vi "PWM Config Pane.vi"(6 "_SubPanelMessages":refnum<notifier>, 9 "_myEmbeddedToFrameEvent":T7, 10 "_myEmbedded.Exit":refnum<user-event>, 11 "-Property Bundle":cluster{"Name":string, "Value":variant}[](array[cluster])) -> (1 "_Connection Informations":T1, 2 "_Scripter Input":T9)   [LabVIEW 2021]
doc: "Generates a pulse width modulation (PWM) signal."
uses:
  <vilib>/myRIO/Common/Express VI Framework/xctls/myRIO Channel Name/myRIO Channel Name.xctl
  <vilib>/myRIO/Common/Express VI Framework/typedefs/Config Pane to Framework Ref.ctl
  <vilib>/myRIO/Common/Express VI Framework/typedefs/Data Validate Ref.ctl
  <vilib>/myRIO/Common/Express VI Framework/typedefs/Scripter Input.ctl
  <vilib>/myRIO/Common/Express VI Framework/typedefs/WireThrough Terminal Names.ctl
  <vilib>/myRIO/Common/Express VI Framework/typedefs/Instrument Driver Method Descriptor Array.ctl
  <vilib>/myRIO/Common/Express VI Framework/typedefs/Instrument Driver Method Descriptor.ctl
  <vilib>/myRIO/Common/Express VI Framework/typedefs/Sub Panel Messages.ctl
  <vilib>/myRIO/Common/Express VI Framework/typedefs/Connection Informations.ctl
  <vilib>/myRIO/Common/Instrument Driver Framework/Utilities/typedefs/Channel Types.ctl
  <vilib>/myRIO/Common/Express VI Framework/vis/Express VI Framework Strings Global.vi
panel:
  out "-Channel Details:":string caption="Connection:"
  in  "Duty Cycle:":dbl(slide)=0.5 min=0.0 max=1.0 step=0.01 scale=0.0..1.0
  out "_learnMoreFrequency":string="Detailed information about valid frequencies for this Express VI.\nLearn more"
  in  "_Validate":bool
  in  "Frequency:":dbl=1000.0 min=0.0 max=400000.0
  in  "Frequency Unit":enum16{"Hz", "kHz"}(ring)
  in  "Duty cycle mode":T2(radio) caption="Duty cycle:"
  in  "Frequency mode":T3(radio) caption="Frequency:"
  out "_Output Preview:":dbl[](graph) caption="Output preview:"
  in  "Channel:":u16(xcontrol)
  in  "_Default Alias String":string
  in  "_VI Default Name (Edit and make value default)":string="PWM"
  in  "Name:":string caption="Node name:"
  in  "_WireThrough Info (Edit and make value default)":T4={"WireThrough Top In"="PWM Ref In", "WireThrough Bottom In"="error in (no error)", "WireThrough Top Out"="PWM Ref Out", "WireThrough Bottom Out"="error out"}
  in  "_Template Array (Edit and make value default)":T5=[{"Function Name"="Smart Open", "VI Path"=path "<vilib>/myRIO/Instrument Drivers/Onboard IO/PWM/vis", "Script"=TRUE, "Inputs"=[{"name"="Channel Name", "value"=variant, "Config Pane Only"=TRUE, "Build Array"=FALSE, "Bundle Cluster"=FALSE, "Show Term"=FALSE, "alias"=[], "Required Input"=FALSE}], "Outputs"=[], "VI Class"=enum."Open", "Controls Refs[]"=[], "Inline"=FALSE}, {"Function Name"="Open", "VI Path"=path "<vilib>/myRIO/Instrument Drivers/Onboard IO/PWM/vis", "Script"=FALSE, "Inputs"=[{"name"="Channel Name", "value"=variant, "Config Pane Only"=TRUE, "Build Array"=FALSE, "Bundle Cluster"=FALSE, "Show Term"=FALSE, "alias"=[], "Required Input"=FALSE}], "Outputs"=[], "VI Class"=enum."Open", "Controls Refs[]"=[], "Inline"=FALSE}, {"Function Name"="Set Duty Cycle and Frequency", "VI Path"=path "<vilib>/myRIO/Instrument Drivers/Onboard IO/PWM/vis", "Script"=TRUE, "Inputs"=[{"name"="Duty Cycle", "value"=variant, "Config Pane Only"=FALSE, "Build Array"=FALSE, "Bundle Cluster"=FALSE, "Show Term"=TRUE, "alias"=[], "Required Input"=TRUE}, {"name"="Frequency [Hz]", "value"=variant, "Config Pane Only"=FALSE, "Build Array"=FALSE, "Bundle Cluster"=FALSE, "Show Term"=TRUE, "alias"=[], "Required Input"=TRUE}], "Outputs"=[], "VI Class"=enum."Data", "Controls Refs[]"=[], "Inline"=FALSE}, {"Function Name"="Close", "VI Path"=path "<vilib>/myRIO/Instrument Drivers/Onboard IO/PWM/vis", "Script"=FALSE, "Inputs"=[], "Outputs"=[], "VI Class"=enum."Close", "Controls Refs[]"=[], "Inline"=FALSE}]
  in  "_Test Close":bool
  # "User Visible Area"
  # "NOTE: Tab Order has been set\nfor this Front Panel.\n\nSee Edit>>Set Tabbing Order...\n\nAll controls that are not visible at \nruntime are excluded from Tabbing order\n\nTo exlude a control from context\nhelp prefix its label text with a '-'"
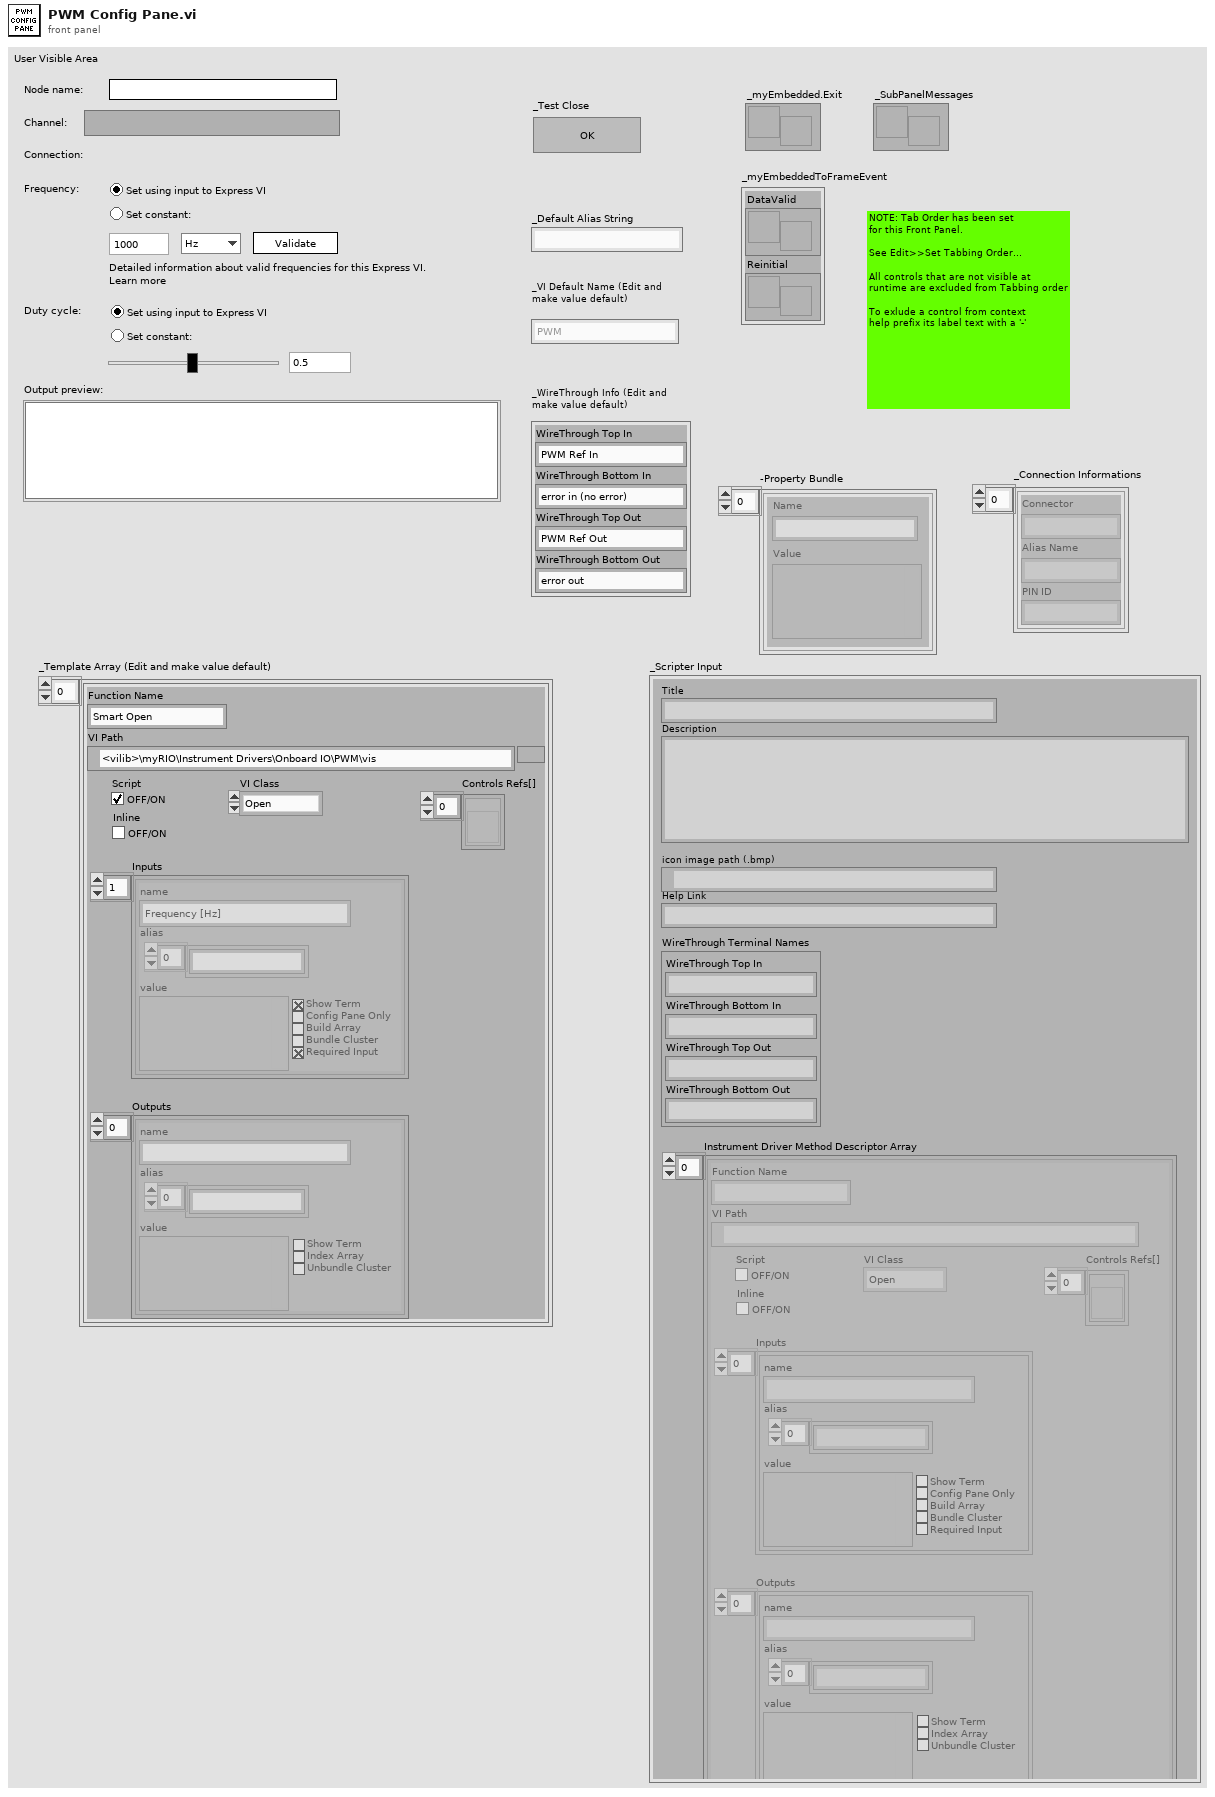
[diagram p1: front panel]
types:
  T1 = typedef "Connection Informations.ctl" = cluster{"Connector":string, "Alias Name":string, "PIN ID":string}[]
  T2 = enum32{"Run-time duty cycle", "Constant duty cycle"}
  T3 = enum32{"Run-time frequency", "Constant frequency"}
  T4 = typedef "WireThrough Terminal Names.ctl" = cluster{"WireThrough Top In":string, "WireThrough Bottom In":string, "WireThrough Top Out":string, "WireThrough Bottom Out":string}
  T5 = typedef "Instrument Driver Method Descriptor Array.ctl" = T6[]
  T6 = typedef "Instrument Driver Method Descriptor.ctl" = cluster{"Function Name":string, "VI Path":path, "Script":bool, "Inputs":cluster{"name":string, "value":variant, "Config Pane Only":bool, "Build Array":bool, "Bundle Cluster":bool, "Show Term":bool, "alias":string[], "Required Input":bool}[], "Outputs":cluster{"name":string, "value":variant, "Show Term":bool, "Index Array":bool, "Unbundle Cluster":bool, "alias":string[]}[], "VI Class":enum16{"Open", "Configure", "Data", "Manage", "Close"}, "Controls Refs[]":refnum<vi>[], "Inline":bool}
  T7 = typedef "Config Pane to Framework Ref.ctl" = cluster{"DataValid":T8, "Reinitial":refnum<user-event>}
  T8 = typedef "Data Validate Ref.ctl" = refnum<user-event>
  T9 = typedef "Scripter Input.ctl" = cluster{"Title":string, "Description":string, "icon image path (.bmp)":path, "Help Link":string, "WireThrough Terminal Names":T4, "Instrument Driver Method Descriptor Array":T5}
  T10 = enum8{"Enabled", "Disabled", "Disabled and Grayed Out"}
  T11 = typedef "Channel Types.ctl" = enum32{"Unknown", "AI", "AO", "DIO - DI", "DIO", "DIO - DO", "I2C", "PWM", "Encoder", "SPI", "UART", "Accelerometer", "DIO - LED", "DIO - Button", "AI (N Samples)", "AudioIn (N Samples)", "AO (N Samples)", "AudioOut (N Samples)", "DI (N Samples)", "DO (N Samples)", "AI IRQ", "DI IRQ", "Timer IRQ", "RSL", "Relay", "CAN", "AI (Continuous)", "AO (Continuous)"}
  T12 = typedef "Channel Info.ctl" = cluster{"Channel Name":string, "Alias":string, "Used?":bool, "Not Support?":bool, "Property Bundle":cluster{"Name":string, "Value":variant}[]}
  T13 = typedef "Sub Panel Messages.ctl" = enum16{"Initialized"}
  T14 = cluster{"Connector":string, "Alias Name":string, "PIN ID":string}
  T15 = cluster{"name":string, "value":variant, "Config Pane Only":bool, "Build Array":bool, "Bundle Cluster":bool, "Show Term":bool, "alias":string[], "Required Input":bool}[]
  T16 = cluster{"name":string, "value":variant, "Config Pane Only":bool, "Build Array":bool, "Bundle Cluster":bool, "Show Term":bool, "alias":string[], "Required Input":bool}
  T17 = cluster{"Connector":string, "Alias Name":string, "PIN ID":string}[]
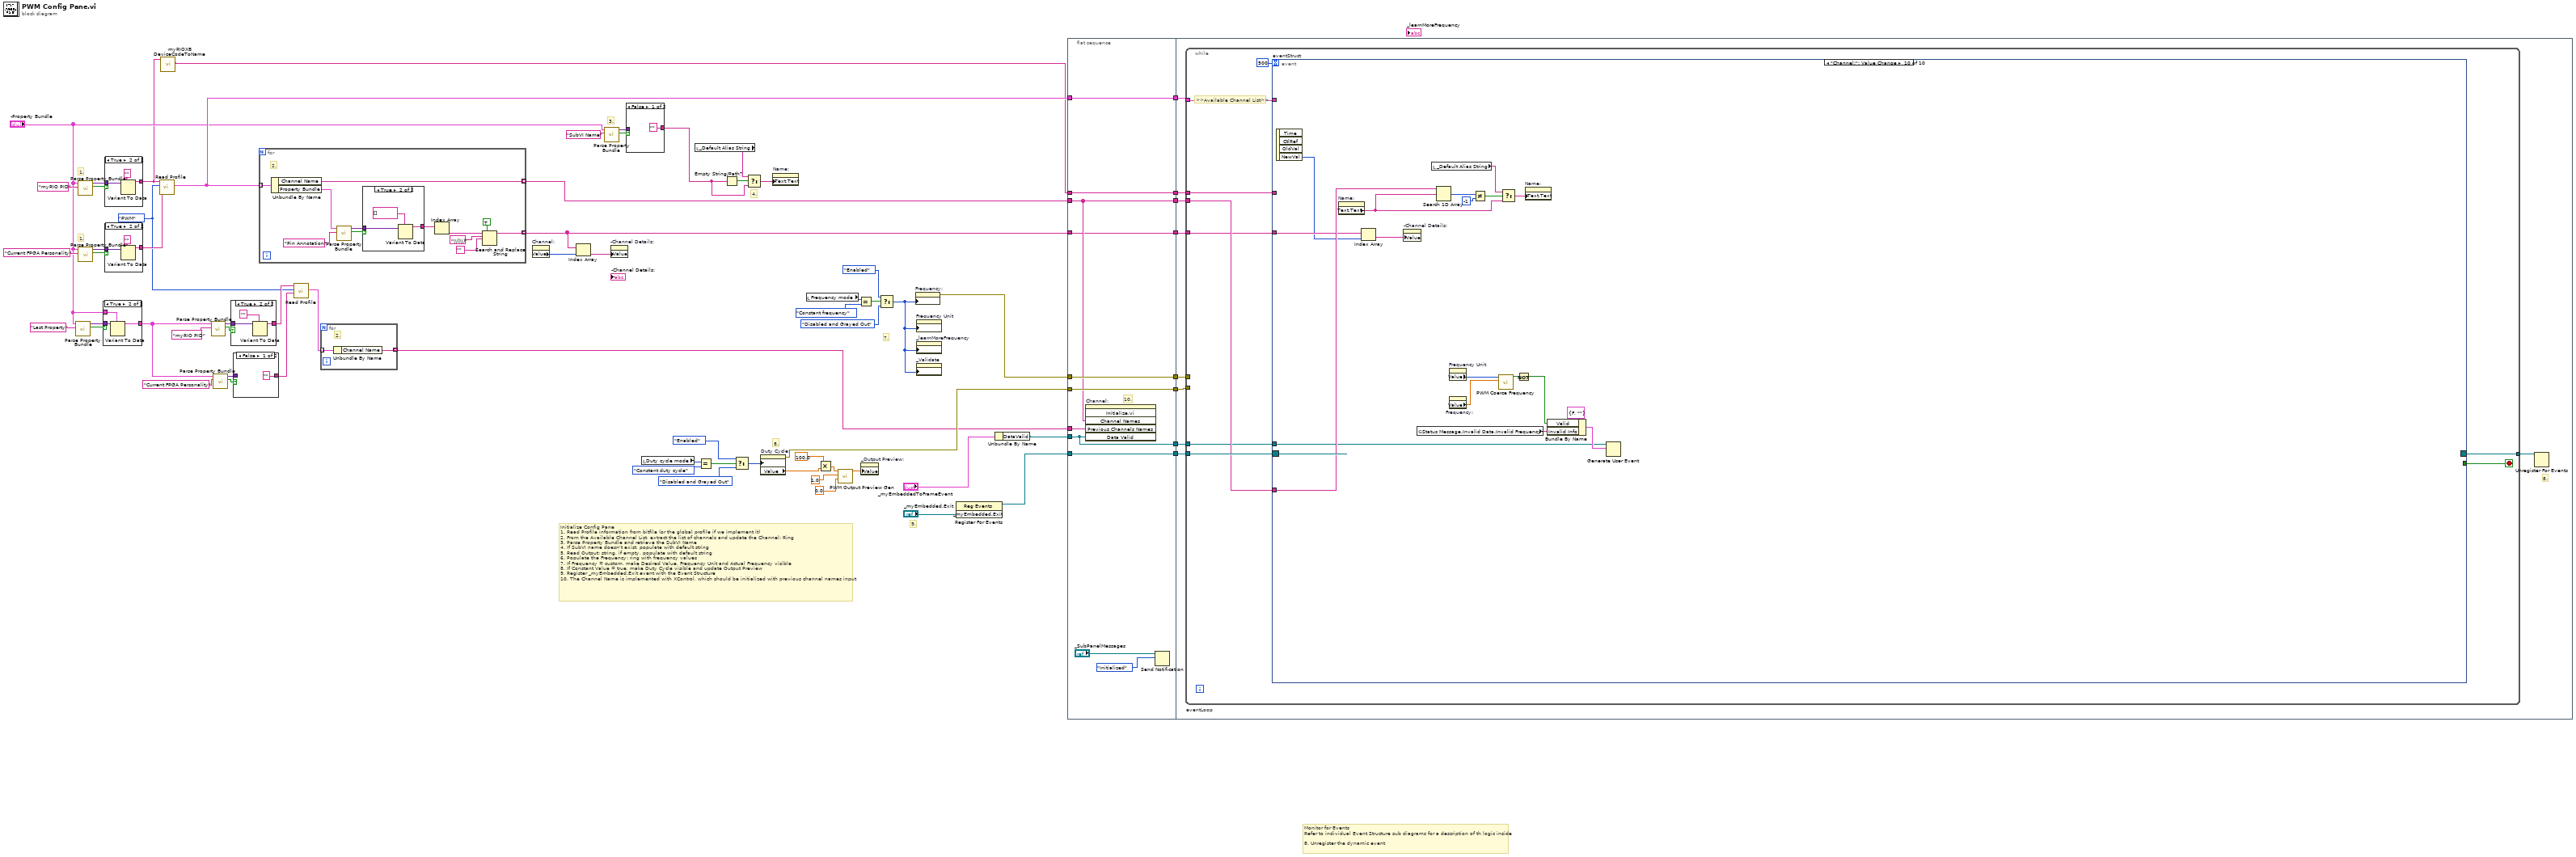
[diagram p0: block diagram]
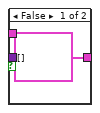
[diagram p2: hidden frame]
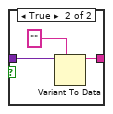
[diagram p3: hidden frame]
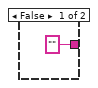
[diagram p4: hidden frame]
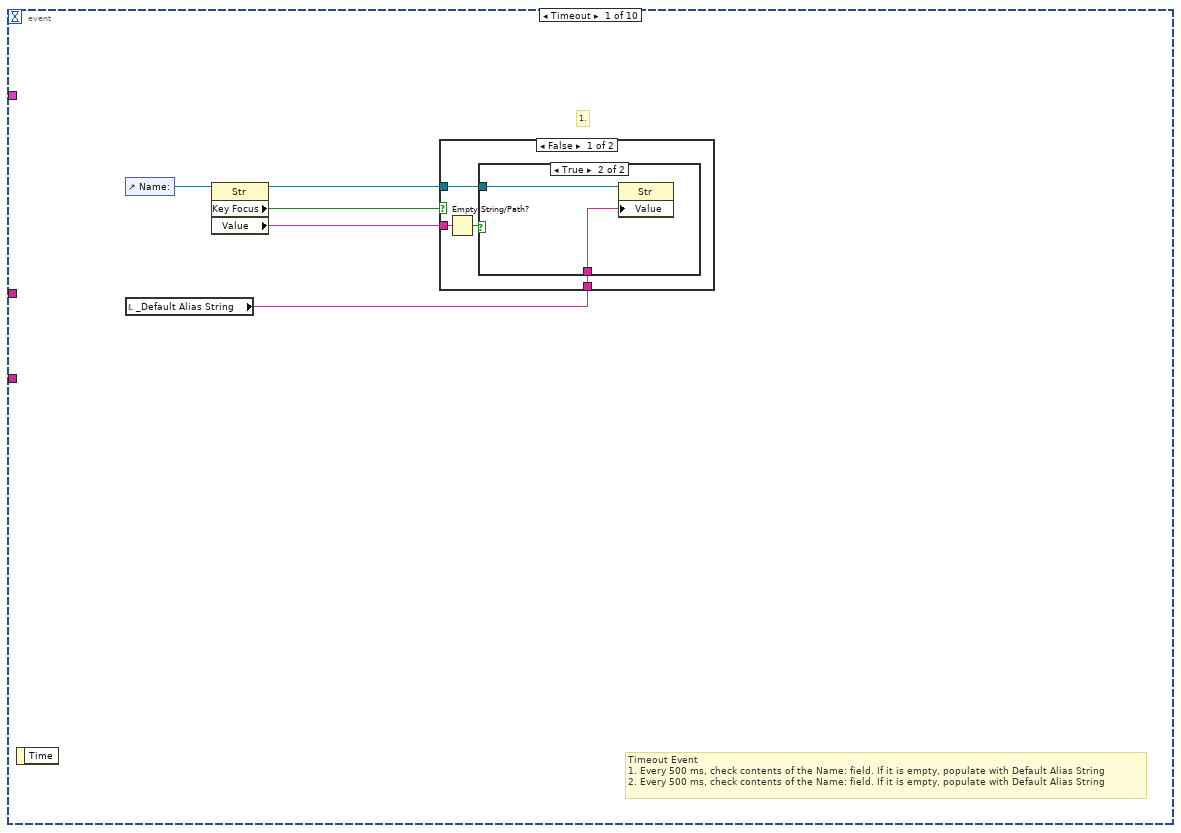
[diagram p5: hidden frame]
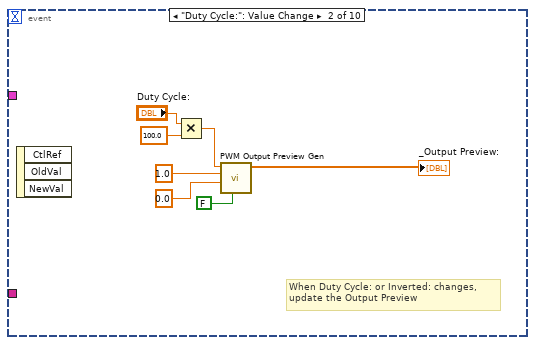
[diagram p8: hidden frame]
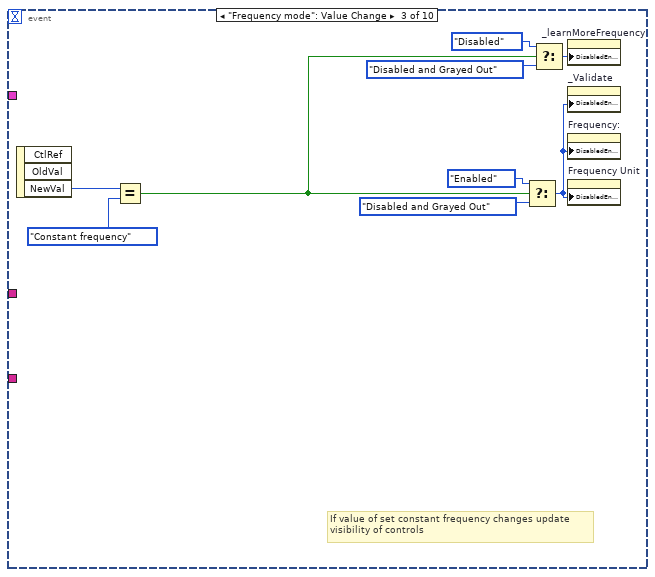
[diagram p9: hidden frame]
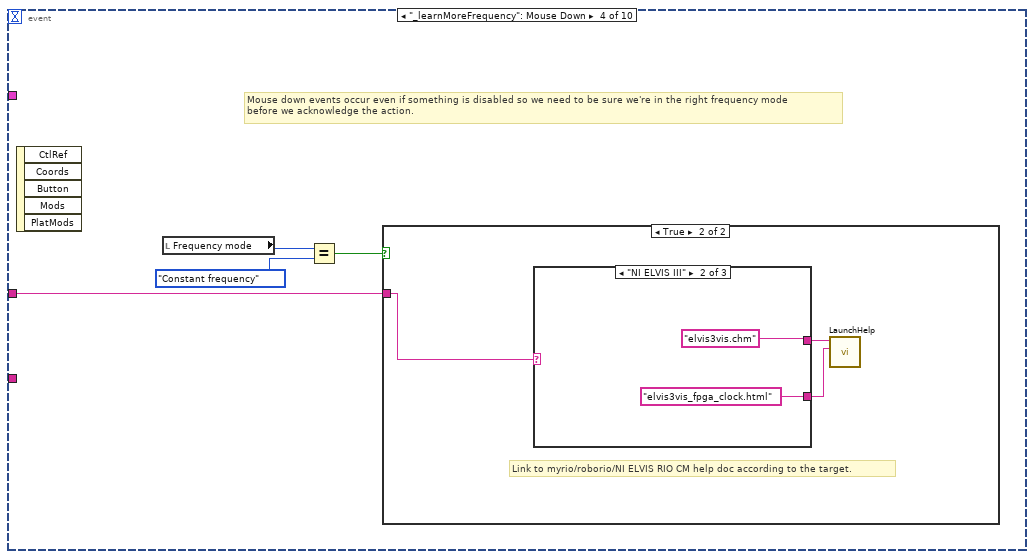
[diagram p10: hidden frame]
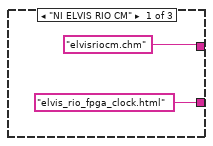
[diagram p12: hidden frame]
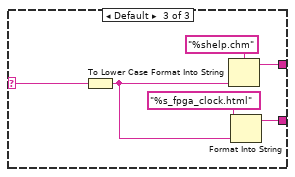
[diagram p13: hidden frame]
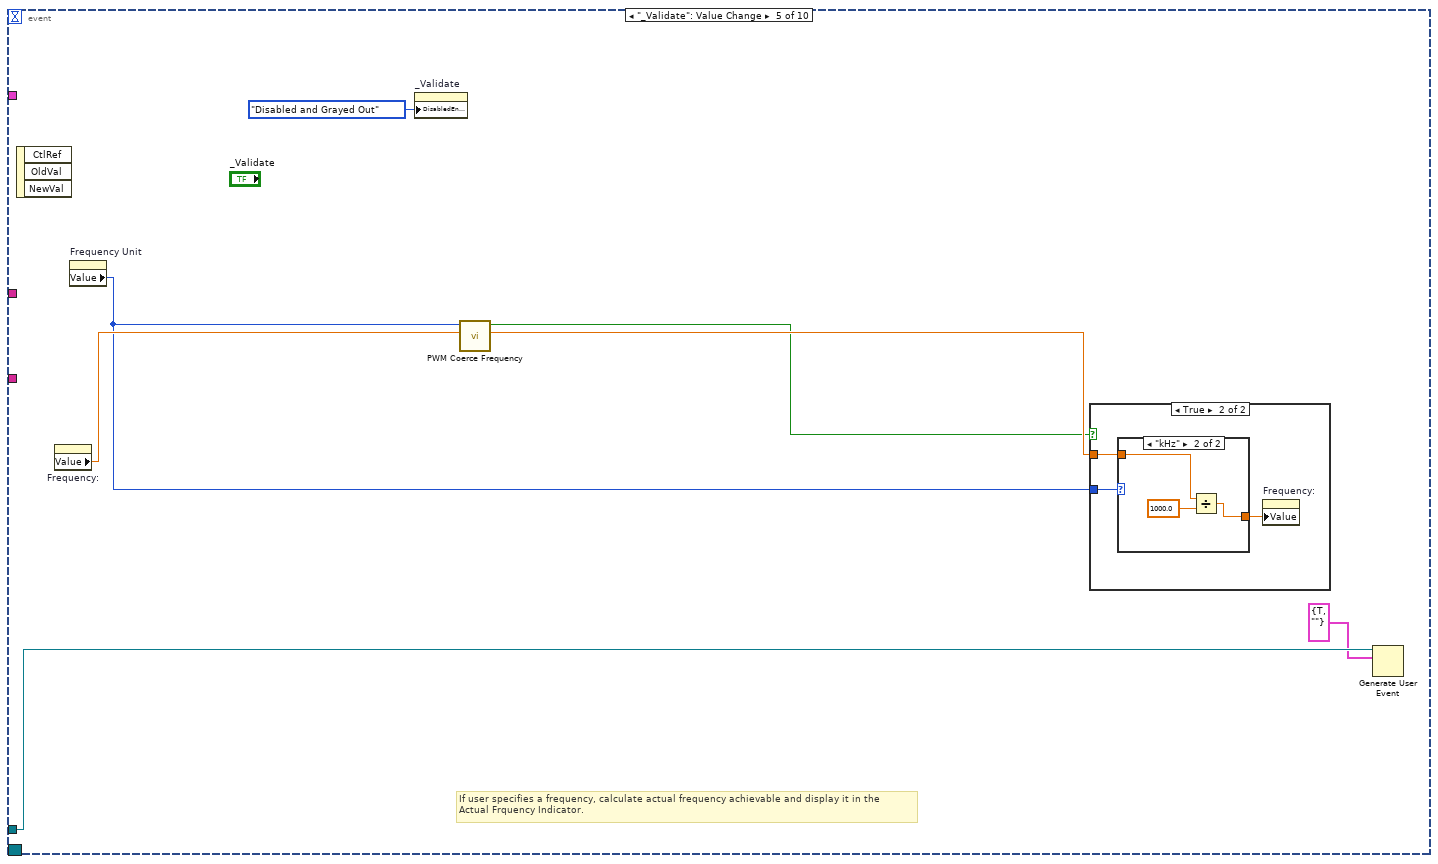
[diagram p14: hidden frame]
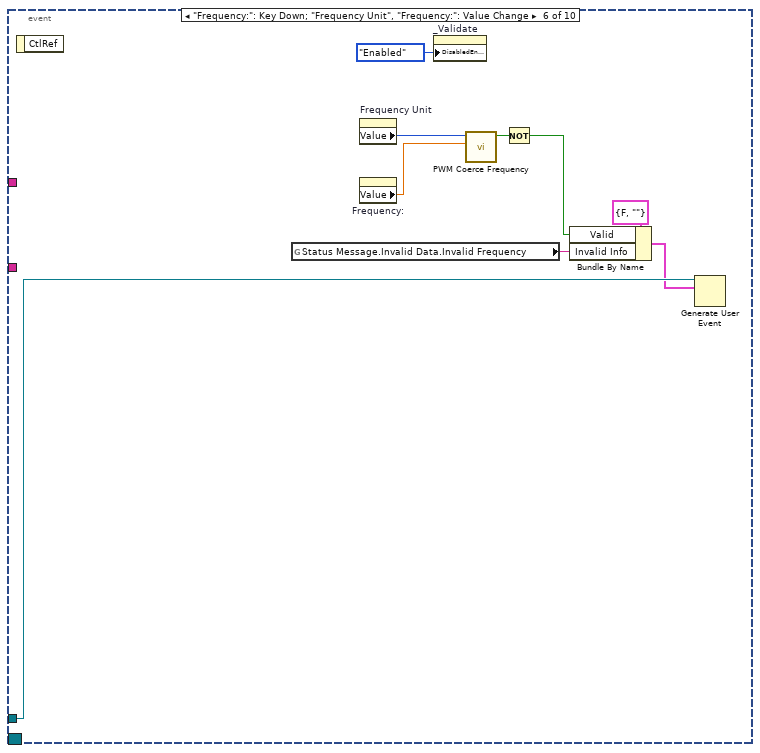
[diagram p17: hidden frame]
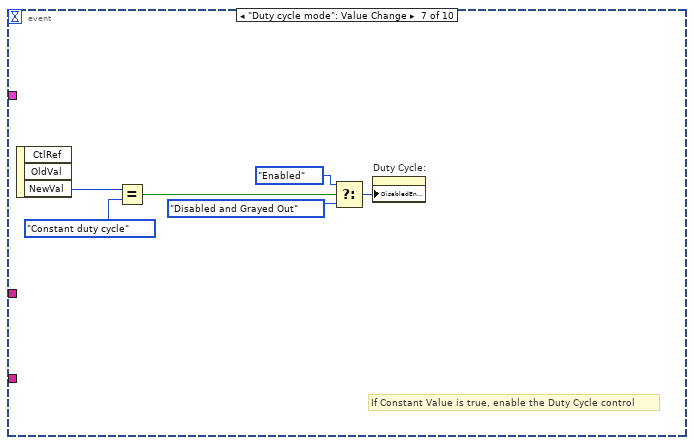
[diagram p18: hidden frame]
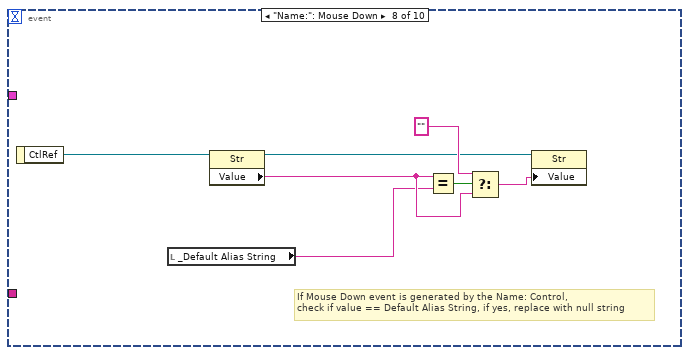
[diagram p19: hidden frame]
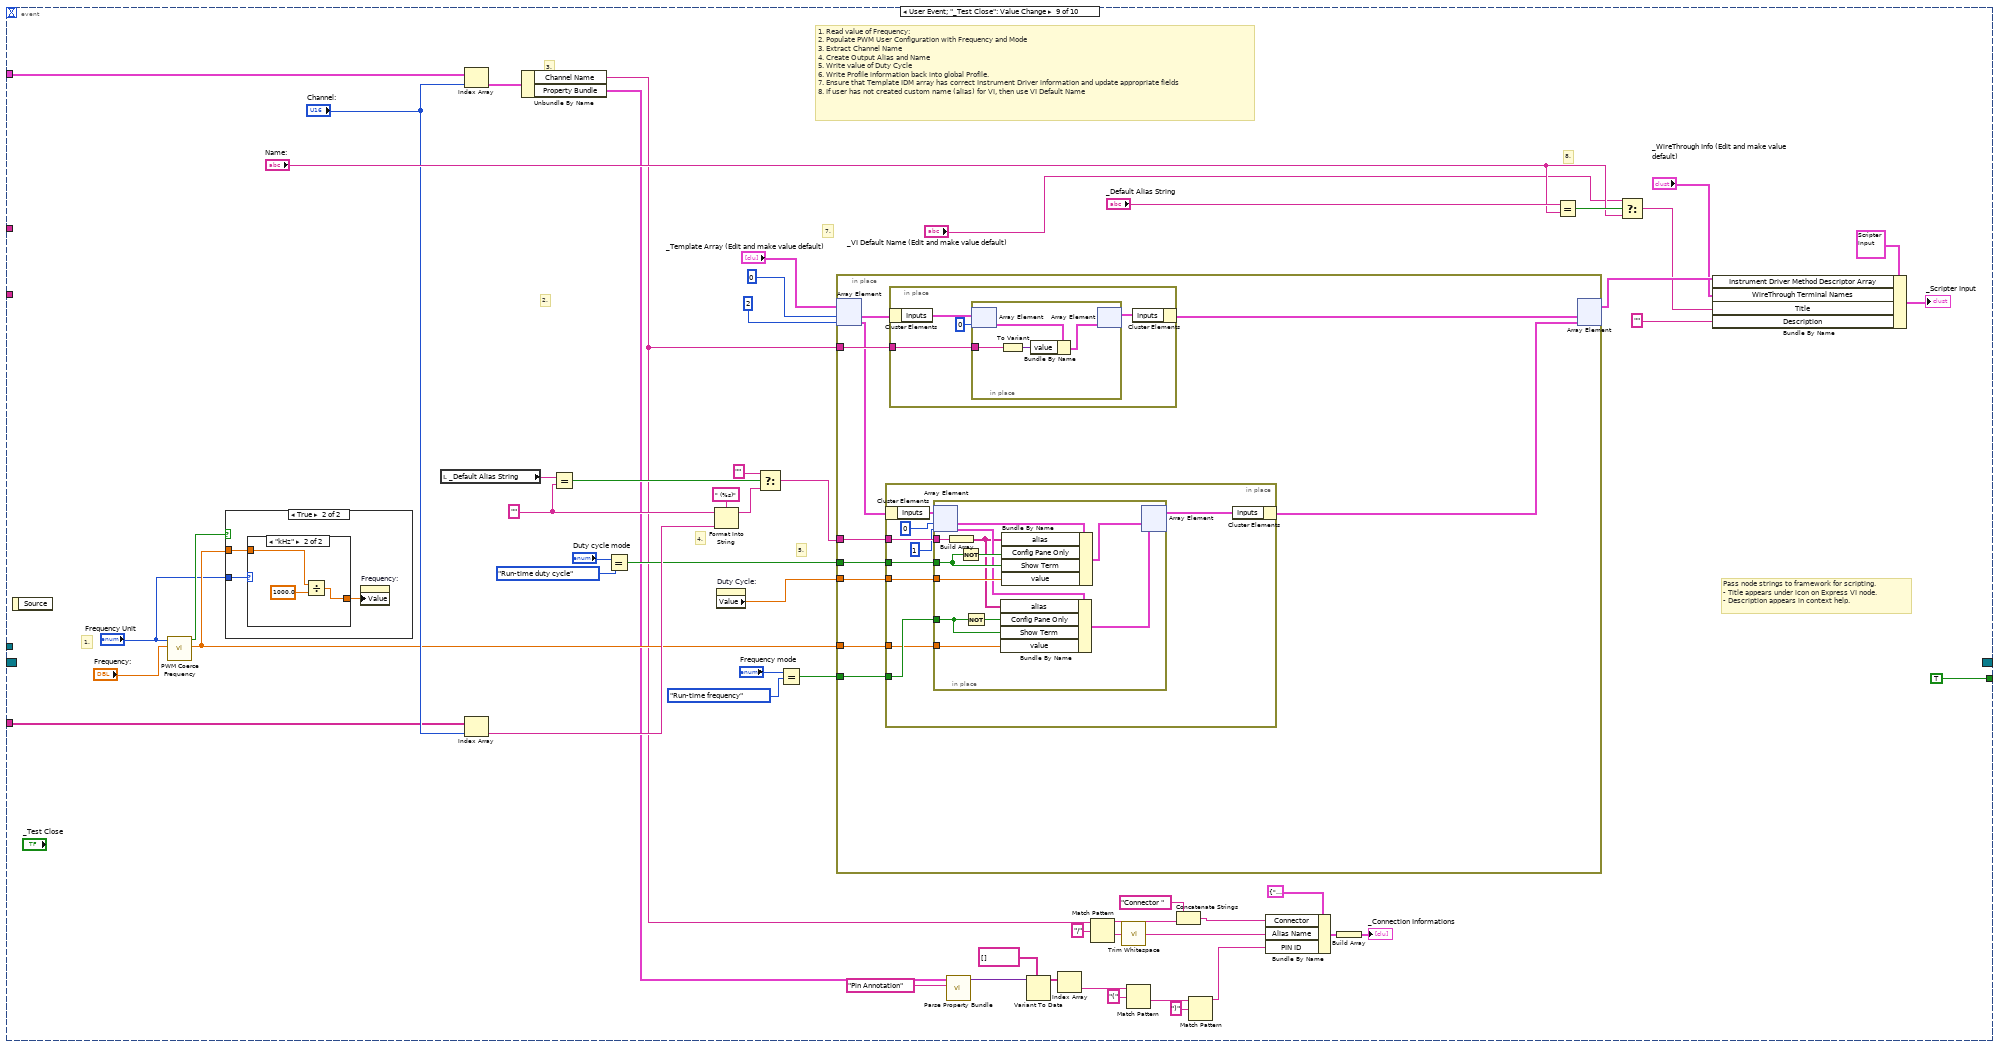
[diagram p20: hidden frame]
diagram:
  w12 = Channel_Types."PWM" ("Channel to Read")
  # "1."
  # "1."
  # "9."
  # "8."
  # "7."
  # "4."
  # "Monitor for Events\nRefer to individual Event Structure sub diagrams for a description of th logic inside\n\n8. Unregister the dynamic event"
  # "3."
  # "Initialize Config Pane\n1. Read Profile information from bitfile (or the global profile if we implement it)\n2. From the Available Channel List, extract the list of channels and update the Channel: Ring\n3. Parse Property Bundle and retrieve the SubVI Name\n4. If SubVI name doesn't exist, populate with default string\n5. Read Output: string, if empty, populate with default string\n6. Populate the Frequency: ring with frequency values\n7. If Frequency = custom, make Desired Value, Frequency Unit and Actual Frequency visible\n8. If Constant Value = true, make Duty Cycle visible and update Output Preview \n9. Register _myEmbedded.Exit event with the Event Structure\n10. The Channel Name is implemented with XControl, which should be initialized with previous channel names input"
  n1 = call <vilib>:"Parse Property Bundle.vi"("Name"="Last Property", "Property Bundle"="-Property Bundle") -> ("Found?"=w15:bool, "Value"=w16:variant)  [unwired: 8 in]
  n2 = call <vilib>:"Parse Property Bundle.vi"("Name"="myRIO PID", "Property Bundle"="-Property Bundle") -> ("Found?"=w51:bool, "Value"=w52:variant)  [unwired: 8 in]
  n3 = call <vilib>:"Parse Property Bundle.vi"("Name"="Current FPGA Personality", "Property Bundle"="-Property Bundle") -> ("Found?"=w35:bool, "Value"=w34:variant)  [unwired: 8 in]
  n4 = case shown="True" w15 {
    tunnel: w16 -> [_ w73]
    tunnel: [cluster{"Name":string, "Value":variant}[] [] ("_Property Bundle") w72] -> w14
    tunnel: "-Property Bundle" -> [_ w71]
    frame False {
    }
    frame True {
      n5 = Variant To Data(type=w71, Variant=w73) -> (data=w72:cluster{"Name":string, "Value":variant}[])  [unwired: 1 in, 1 out]
    }
  }
  n6 = case shown="True" w51 {
    tunnel: w52 -> [_ w77]
    tunnel: ["" ("Name") w75] -> w5
    frame False {
    }
    frame True {
      n7 = Variant To Data(type="" ("Name"), Variant=w77) -> (data=w75:string)  [unwired: 1 in, 1 out]
    }
  }
  n8 = case shown="True" w35 {
    tunnel: w34 -> [_ w81]
    tunnel: ["" ("Name") w79] -> w32
    frame False {
    }
    frame True {
      n9 = Variant To Data(type="" ("Name"), Variant=w81) -> (data=w79:string)  [unwired: 1 in, 1 out]
    }
  }
  n10 = call <vilib>:"Read Profile.vi"("FPGA Name"=w32, "Channel to Read"=w12, "myRIO PID"=w5) -> ("Channel List Out"=w50:T12[])  [unwired: 7 in, 1 out]
  n11 = call <vilib>:"myRIOXB DeviceCodeToName.vi"("Device Code"=w5) -> ("Name"=w6:string)  [unwired: 10 in]
  n12 = call <vilib>:"Parse Property Bundle.vi"("Name"="myRIO PID", "Property Bundle"=w14) -> ("Found?"=w24:bool, "Value"=w23:variant)  [unwired: 8 in]
  n13 = call <vilib>:"Parse Property Bundle.vi"("Name"="Current FPGA Personality", "Property Bundle"=w14) -> ("Found?"=w19:bool, "Value"=w20:variant)  [unwired: 8 in]
  n14 = case shown="True" w24 {
    tunnel: w23 -> [_ w85]
    tunnel: ["" ("Name") w83] -> w25
    frame False {
    }
    frame True {
      n15 = Variant To Data(type="" ("Name"), Variant=w85) -> (data=w83:string)  [unwired: 1 in, 1 out]
    }
  }
  n16 = case shown="False" w19 {
    tunnel: w20 -> [_ w89]
    tunnel: ["" ("Name") w87] -> w18
    frame False {
    }
    frame True {
      n17 = Variant To Data(type="" ("Name"), Variant=w89) -> (data=w87:string)  [unwired: 1 in, 1 out]
    }
  }
  n18 = for {
    tunnel: w50 -> [w101] mode=indexing
    tunnel: [w95] -> w31 mode=indexing
    tunnel: [w93] -> w2 mode=indexing
    # "2."
    n19 = Unbundle By Name(w101) -> ("Channel Name"=w95:string, "Property Bundle"=w100:cluster{"Name":string, "Value":variant}[])
    n20 = call <vilib>:"Parse Property Bundle.vi"("Name"="Pin Annotation", "Property Bundle"=w100) -> ("Found?"=w97:bool, "Value"=w98:variant)  [unwired: 8 in]
    n21 = case shown="True" w97 {
      tunnel: w98 -> [_ w105]
      tunnel: [string[] [] w104] -> w96
      frame False {
      }
      frame True {
        n22 = Variant To Data(type=string[] [], Variant=w105) -> (data=w104:string[])  [unwired: 1 in, 1 out]
      }
    }
    n23 = Index Array(array=w96) -> (element=w94:string)  [unwired: 1 in]
    n24 = Search and Replace String(replace all?=TRUE ("replace all? (F)"), input string=w94, search string="\\(|\\)", replace string="") -> (result string=w93:string)  [unwired: 4 in, 3 out]
  }
  n25 = call <vilib>:"Read Profile.vi"("FPGA Name"=w18, "Channel to Read"=w12, "myRIO PID"=w25) -> ("Channel List Out"=w11:T12[])  [unwired: 7 in, 1 out]
  n26 = for {
    tunnel: w11 -> [w107] mode=indexing
    tunnel: [w106] -> w10 mode=indexing
    # "2."
    n27 = Unbundle By Name(w107) -> ("Channel Name"=w106:string)
  }
  n28 = property on="Channel:" class="myRIO Channel Name (strict)"() -> ("Value"=w4:u16)  [unwired: 2 in, 2 out]
  n29 = Index Array(array=w2, index=w4) -> (element=w1:string)
  n30 = call <vilib>:"Parse Property Bundle.vi"("Name"="SubVI Name", "Property Bundle"="-Property Bundle") -> ("Found?"=w56:bool, "Value"=w55:variant)  [unwired: 8 in]
  n31 = property on="-Channel Details:" class="Str"("Value"=w1) -> ()  [unwired: 2 in, 2 out]
  n32 = case shown="False" w56 {
    tunnel: w55 -> [_ w111]
    tunnel: ["" ("Name") w109] -> w54
    frame False {
    }
    frame True {
      n33 = Variant To Data(type="" ("Name"), Variant=w111) -> (data=w109:string)  [unwired: 1 in, 1 out]
    }
  }
  n34 = local read "Duty cycle mode"() -> (w39:T2)
  n35 = local read "_Default Alias String"() -> (w64:string)
  n36 = Equal?(x=w39, y=T2."Constant duty cycle") -> (x = y?=w37:bool)
  n37 = Empty String/Path?(string/path=w54) -> (empty?=w66:bool)
  n38 = Select(t=T10."Enabled" ("Disabled"), s=w37, f=T10."Disabled and Grayed Out" ("Disabled")) -> (s? t:f=w61:T10)
  n39 = Select(t=w64, s=w66, f=w54) -> (s? t:f=w65:string)
  n40 = property on="Duty Cycle:" class="Slide (strict)"("DisabledEnum"=w61) -> (error out=w43:errorcluster, "Value"=w48:dbl)  [unwired: 2 in, 1 out]
  n41 = property on="Name:" class="Str"("Text.Text"=w65) -> ()  [unwired: 2 in, 2 out]
  n42 = local read "Frequency mode"() -> (w42:T3)
  n43 = Multiply(x=100.0, y=w48) -> (x*y=w49:dbl)
  n44 = call <vilib>:"PWM Output Preview Gen.vi"("Low Level"=0.0 ("element"), "High Level"=1.0 ("element"), "Duty Cycle (4-96%)"=w49) -> ("Output Array"=w58:dbl[])  [unwired: 8 in]
  n45 = Equal?(x=w42, y=T3."Constant frequency") -> (x = y?=w40:bool)
  n46 = property on="_Output Preview:" class="WFGraph (strict)"("Value"=w58) -> ()  [unwired: 2 in, 2 out]
  n47 = Select(t=T10."Enabled" ("Disabled"), s=w40, f=T10."Disabled and Grayed Out" ("Disabled")) -> (s? t:f=w36:T10)
  n48 = property on="Frequency:" class="DigNum (strict)"("DisabledEnum"=w36) -> (error out=w44:errorcluster)  [unwired: 2 in, 1 out]
  n49 = property on="Frequency Unit" class="Enum (strict)"("DisabledEnum"=w36) -> ()  [unwired: 2 in, 2 out]
  n50 = property on="_learnMoreFrequency" class="Str"("DisabledEnum"=w36) -> ()  [unwired: 2 in, 2 out]
  n51 = property on="_Validate" class="Bool"("DisabledEnum"=w36) -> ()  [unwired: 2 in, 2 out]
  n52 = register-events("_myEmbedded.Exit") -> (reference out=w69:refnum<event-registration>)  [unwired: 2 in, 1 out]
  n53 = Unbundle By Name("_myEmbeddedToFrameEvent") -> ("DataValid"=w9:T8)
  n54 = flat-sequence {
    tunnel: w9 -> [w113]
    tunnel: w31 -> [w115]
    tunnel: w43 -> [w119]
    tunnel: w44 -> [w120]
    tunnel: w50 -> [w121]
    tunnel: w69 -> [w122]
    tunnel: [w122] -> w30
    tunnel: [w121] -> w29
    tunnel: [w120] -> w28
    tunnel: [w119] -> w27
    tunnel: [w115] -> w26
    tunnel: w10 -> [w116]
    tunnel: w6 -> [w114]
    tunnel: [w114] -> w8
    tunnel: [w113] -> w7
    tunnel: w2 -> [w112]
    tunnel: [w112] -> w3
    tunnel: w30 -> [w131]
    tunnel: w29 -> [w129]
    tunnel: w28 -> [w128]
    tunnel: w27 -> [w127]
    tunnel: w26 -> [w126]
    tunnel: w8 -> [w125]
    tunnel: w7 -> [w124]
    tunnel: w3 -> [w123]
    frame #0 {
      # "10."
      n55 = invoke on="Channel:" class="myRIO Channel Name (strict)" method="Initialize.vi"("Channel Names"=w115, "Previous Channels Names"=w116, "Data Valid"=w113) -> ()  [unwired: 3 in, 6 out]
      n56 = Send Notification(notification=Sub_Panel_Messages."Initialized", notifier="_SubPanelMessages") -> ()  [unwired: 1 in, 2 out]
    }
    frame #1 {
      # "8."
      n57 = while "eventLoop" {
        tunnel: w131 -> [w139]
        tunnel: [w138] -> w130
        tunnel: w129 -> [w136]
        tunnel: w126 -> [w135]
        tunnel: w128 -> [_]
        tunnel: w127 -> [_]
        tunnel: w125 -> [w134]
        tunnel: w124 -> [w133]
        tunnel: w123 -> [w132]
        stop <- w140 stop-if-true
        # ">>Available Channel List>>"
        n58 = event "eventStruct" shown="[9] \"Channel:\": Value Change" {
          selector: w139 -> [_ _ _ _ _ _ _ _ _ _]
          dyn-events: [_ _ _ _ _ _ _ _ _ _] -> w138
          timeout: 500 -> [_ _ _ _ _ _ _ _ _ _]
          tunnel: [_ _ _ _ _ _ _ _ TRUE ("_Test Close") _] -> w140
          tunnel: w136 -> [_ _ _ _ _ _ _ _ w276 _]
          tunnel: w135 -> [_ _ _ _ _ _ _ _ w252 w335]
          tunnel: w134 -> [_ _ _ w168 _ _ _ _ _ _]
          tunnel: w133 -> [_ _ _ _ w186 w206 _ _ _ w327]
          tunnel: w132 -> [_ _ _ _ _ _ _ _ _ w326]
          event Timeout {
            # "Timeout Event\n1. Every 500 ms, check contents of the Name: field. If it is empty, populate with Default Alias String\n2. Every 500 ms, check contents of the Name: field. If it is empty, populate with Default Alias String"
            # "1."
            n59 = event-data() -> ()  [unwired: 1 in, 1 out]
            n60 = control-ref of="Name:"() -> (w143:refnum<vi>)
            n61 = local read "_Default Alias String"() -> (w141:string)
            n62 = property on="Property Node" class="Str"(reference=w143) -> (reference out=w142:refnum<vi>, "Key Focus"=w144:bool, "Value"=w145:string)  [unwired: 1 in, 1 out]
            n63 = case shown="False" w144 {
              tunnel: w145 -> [w149 _]
              tunnel: w142 -> [w147 _]
              tunnel: w141 -> [w146 _]
              frame False {
                n64 = Empty String/Path?(string/path=w149) -> (empty?=w148:bool)
                n65 = case shown="True" w148 {
                  tunnel: w147 -> [_ w151]
                  tunnel: w146 -> [_ w150]
                  frame False {
                  }
                  frame True {
                    n66 = property on="Property Node" class="Str"(reference=w151, "Value"=w150) -> ()  [unwired: 1 in, 2 out]
                  }
                }
              }
              frame True {
              }
            }
          }
          event "Duty Cycle:": Value Change {
            # "When Duty Cycle: or Inverted: changes, \nupdate the Output Preview"
            n67 = event-data() -> ()  [unwired: 1 in, 3 out]
            n68 = Multiply(x="Duty Cycle:", y=100.0) -> (x*y=w153:dbl)
            n69 = call <vilib>:"PWM Output Preview Gen.vi"("Invert"=FALSE, "Low Level"=0.0 ("element"), "High Level"=1.0 ("element"), "Duty Cycle (4-96%)"=w153) -> ("Output Array"=→"_Output Preview:":dbl[])  [unwired: 7 in]
          }
          event "Frequency mode": Value Change {
            # "If value of set constant frequency changes update\nvisibility of controls"
            n70 = event-data() -> ("NewVal"=w165:T3)  [unwired: 1 in, 2 out]
            n71 = Equal?(x=w165, y=T3."Constant frequency") -> (x = y?=w161:bool)
            n72 = Select(t=T10."Enabled" ("Disabled"), s=w161, f=T10."Disabled and Grayed Out" ("Disabled")) -> (s? t:f=w163:T10)
            n73 = Select(t=T10."Disabled" ("Disabled"), s=w161, f=T10."Disabled and Grayed Out" ("Disabled")) -> (s? t:f=w160:T10)
            n74 = property on="_learnMoreFrequency" class="Str"("DisabledEnum"=w160) -> ()  [unwired: 2 in, 2 out]
            n75 = property on="_Validate" class="Bool"("DisabledEnum"=w163) -> ()  [unwired: 2 in, 2 out]
            n76 = property on="Frequency:" class="DigNum (strict)"("DisabledEnum"=w163) -> ()  [unwired: 2 in, 2 out]
            n77 = property on="Frequency Unit" class="Enum (strict)"("DisabledEnum"=w163) -> ()  [unwired: 2 in, 2 out]
          }
          event "_learnMoreFrequency": Mouse Down {
            # "Mouse down events occur even if something is disabled so we need to be sure we're in the right frequency mode\nbefore we acknowledge the action."
            n78 = event-data() -> ()  [unwired: 1 in, 5 out]
            n79 = local read "Frequency mode"() -> (w171:T3)
            n80 = Equal?(x=w171, y=T3."Constant frequency") -> (x = y?=w169:bool)
            n81 = case shown="True" w169 {
              tunnel: w168 -> [_ w172]
              frame False {
              }
              frame True {
                # "Link to myrio/roborio/NI ELVIS RIO CM help doc according to the target."
                n82 = case shown="\"NI ELVIS III\"" w172 {
                  selector: w172 -> [_ _ w179]
                  tunnel: ["elvisriocm.chm" ("Help File") "elvis3vis.chm" ("Help File") w181] -> w174
                  tunnel: ["elvis_rio_fpga_clock.html" ("Help Topic") "elvis3vis_fpga_clock.html" ("Help Topic") w180] -> w173
                  frame "NI ELVIS RIO CM" {
                  }
                  frame "NI ELVIS III" {
                  }
                  frame Default {
                    n83 = To Lower Case(string=w179) -> (all lower case string=w183:string)
                    n84 = Format Into String(format string="%shelp.chm" ("Help File"), w183) -> (resulting string=w181:string)  [unwired: 2 in, 1 out]
                    n85 = Format Into String(format string="%s_fpga_clock.html" ("Help Topic"), w183) -> (resulting string=w180:string)  [unwired: 2 in, 1 out]
                  }
                }
                n86 = call <vilib>:"LaunchHelp.vi"("Help Topic"=w173, "Help File"=w174) -> ()  [unwired: 10 in]
              }
            }
          }
          event "_Validate": Value Change {
            # "If user specifies a frequency, calculate actual frequency achievable and display it in the \nActual Frquency Indicator."
            n87 = event-data() -> ()  [unwired: 1 in, 3 out]
            n88 = property on="Frequency:" class="DigNum (strict)"() -> ("Value"=w191:dbl)  [unwired: 2 in, 2 out]
            n89 = property on="Frequency Unit" class="Enum (strict)"() -> ("Value"=w190:enum16{"Hz", "kHz"})  [unwired: 2 in, 2 out]
            n90 = property on="_Validate" class="Bool"("DisabledEnum"=T10."Disabled and Grayed Out" ("Disabled")) -> ()  [unwired: 2 in, 2 out]
            n91 = call <vilib>:"PWM Coerce Frequency.vi"("Frequency"=w191, "Frequency Units"=w190) -> ("Coerced Frequency"=w189:dbl, "Coercion needed?"=w188:bool)  [unwired: 8 in]
            n92 = case shown="True" w188 {
              tunnel: w190 -> [_ w194]
              tunnel: w189 -> [_ w193]
              frame False {
              }
              frame True {
                n93 = case shown="\"kHz\"" w194 {
                  tunnel: w193 -> [w195 w198]
                  tunnel: [w195 w196] -> w192
                  frame "Hz", Default {
                  }
                  frame "kHz" {
                    n94 = Divide(x=w198, y=1000.0) -> (x/y=w196:dbl)
                  }
                }
                n95 = property on="Frequency:" class="DigNum (strict)"("Value"=w192) -> ()  [unwired: 2 in, 2 out]
              }
            }
            n96 = Generate User Event(user event=w186, event data cluster=cluster{"Valid":bool, "Invalid Info":string} {"Valid"=TRUE, "Invalid Info"=""} ("event data")) -> ()  [unwired: 2 in, 2 out]
          }
          event "Frequency:": Key Down; "Frequency Unit", "Frequency:": Value Change {
            n97 = event-data() -> ()  [unwired: 1 in, 1 out]
            n98 = global read "Express VI Framework Strings Global.vi" "Status Message.Invalid Data.Invalid Frequency"() -> (w199:string)
            n99 = property on="Frequency Unit" class="Enum (strict)"() -> ("Value"=w203:enum16{"Hz", "kHz"})  [unwired: 2 in, 2 out]
            n100 = property on="Frequency:" class="DigNum (strict)"() -> ("Value"=w202:dbl)  [unwired: 2 in, 2 out]
            n101 = property on="_Validate" class="Bool"("DisabledEnum"=T10."Enabled" ("Disabled")) -> ()  [unwired: 2 in, 2 out]
            n102 = call <vilib>:"PWM Coerce Frequency.vi"("Frequency"=w202, "Frequency Units"=w203) -> ("Coercion needed?"=w201:bool)  [unwired: 8 in, 1 out]
            n103 = Not(x=w201) -> (.not. x?=w200:bool)
            n104 = Bundle By Name(cluster=cluster{"Valid":bool, "Invalid Info":string} {"Valid"=FALSE, "Invalid Info"=""} ("event data"), "Valid"=w200, "Invalid Info"=w199) -> (w204:cluster{"Valid":bool, "Invalid Info":string})
            n105 = Generate User Event(user event=w206, event data cluster=w204) -> ()  [unwired: 2 in, 2 out]
          }
          event "Duty cycle mode": Value Change {
            # "If Constant Value is true, enable the Duty Cycle control"
            n106 = event-data() -> ("NewVal"=w210:T2)  [unwired: 1 in, 2 out]
            n107 = Equal?(x=w210, y=T2."Constant duty cycle") -> (x = y?=w208:bool)
            n108 = Select(t=T10."Enabled" ("Disabled"), s=w208, f=T10."Disabled and Grayed Out" ("Disabled")) -> (s? t:f=w213:T10)
            n109 = property on="Duty Cycle:" class="Slide (strict)"("DisabledEnum"=w213) -> ()  [unwired: 2 in, 2 out]
          }
          event "Name:": Mouse Down {
            # "If Mouse Down event is generated by the Name: Control,\ncheck if value == Default Alias String, if yes, replace with null string"
            n110 = event-data() -> ("CtlRef"=w220:refnum<vi>)  [unwired: 1 in]
            n111 = local read "_Default Alias String"() -> (w214:string)
            n112 = property class="Str"(reference=w220) -> (reference out=w216:refnum<vi>, "Value"=w215:string)  [unwired: 1 in, 1 out]
            n113 = Equal?(x=w215, y=w214) -> (x = y?=w219:bool)
            n114 = Select(t="", s=w219, f=w215) -> (s? t:f=w217:string)
            n115 = property class="Str"(reference=w216, "Value"=w217) -> ()  [unwired: 1 in, 2 out]
          }
          event User Event; "_Test Close": Value Change {
            w256 = "" ("y")
            # "3."
            # "5."
            # "4."
            # "2."
            # "1. Read value of Frequency:\n2. Populate PWM User Configuration with Frequency and Mode\n3. Extract Channel Name\n4. Create Output Alias and Name\n5. Write value of Duty Cycle\n6. Write Profile information back into global Profile.\n7. Ensure that Template IDM array has correct Instrument Driver information and update appropriate fields\n8. If user has not created custom name (alias) for VI, then use VI Default Name"
            # "8."
            # "7."
            # "1."
            # "Pass node strings to framework for scripting.\n- Title appears under icon on Express VI node.\n- Description appears in context help."
            n116 = event-data() -> ()  [unwired: 1 in, 1 out]
            n117 = call <vilib>:"PWM Coerce Frequency.vi"("Frequency"="Frequency:", "Frequency Units"="Frequency Unit") -> ("Coerced Frequency"=w243:dbl, "Coercion needed?"=w242:bool)  [unwired: 8 in]
            n118 = case shown="True" w242 {
              tunnel: "Frequency Unit" -> [_ w280]
              tunnel: w243 -> [_ w279]
              frame False {
              }
              frame True {
                n119 = case shown="\"kHz\"" w280 {
                  tunnel: w279 -> [w281 w284]
                  tunnel: [w281 w282] -> w278
                  frame "Hz", Default {
                  }
                  frame "kHz" {
                    n120 = Divide(x=w284, y=1000.0) -> (x/y=w282:dbl)
                  }
                }
                n121 = property on="Frequency:" class="DigNum (strict)"("Value"=w278) -> ()  [unwired: 2 in, 2 out]
              }
            }
            n122 = local read "_Default Alias String"() -> (w261:string)
            n123 = Index Array(array=w276, index="Channel:") -> (element=w254:T12)
            n124 = Index Array(array=w252, index="Channel:") -> (element=w251:string)
            n125 = Unbundle By Name(w254) -> ("Channel Name"=w228:string, "Property Bundle"=w227:cluster{"Name":string, "Value":variant}[])
            n126 = Equal?(x=w261, y=w256) -> (x = y?=w264:bool)
            n127 = Equal?(x="Duty cycle mode", y=T2."Run-time duty cycle") -> (x = y?=w248:bool)
            n128 = Format Into String(format string=" (%s)", initial string=w256, w251) -> (resulting string=w262:string)  [unwired: 1 in, 1 out]
            n129 = property on="Duty Cycle:" class="Slide (strict)"() -> ("Value"=w257:dbl)  [unwired: 2 in, 2 out]
            n130 = Select(t="", s=w264, f=w262) -> (s? t:f=w259:string)
            n131 = Equal?(x="Frequency mode", y=T3."Run-time frequency") -> (x = y?=w245:bool)
            n132 = in-place {
              in-place-border: w228 -> [w292]
              in-place-border: w259 -> [w291]
              in-place-border: w257 -> [w290]
              in-place-border: w243 -> [w289]
              in-place-border: w248 -> [w286]
              in-place-border: w245 -> [w285]
              n133 = in-place-array #1("_Template Array (Edit and make value default)", 0, 2) -> (w294:T6, w288:T6)
              n134 = in-place {
                in-place-border: w291 -> [w300]
                in-place-border: w290 -> [w302]
                in-place-border: w289 -> [w295]
                in-place-border: w286 -> [w299]
                in-place-border: w285 -> [w296]
                n135 = in-place-cluster #2(w288) -> ("Inputs"=w301:T15)
                n136 = in-place {
                  in-place-border: w300 -> [w313]
                  in-place-border: w302 -> [w312]
                  in-place-border: w299 -> [w310]
                  in-place-border: w296 -> [w305]
                  in-place-border: w295 -> [w304]
                  n137 = in-place-array #3(w301, 0, 1) -> (w315:T16, w308:T16)
                  n138 = Build Array(w313) -> (w306:string[])
                  n139 = Not(x=w310) -> (.not. x?=w311:bool)
                  n140 = Not(x=w305) -> (.not. x?=w309:bool)
                  n141 = Bundle By Name(cluster=w308, "alias"=w306, "Config Pane Only"=w309, "Show Term"=w305, "value"=w304) -> (w307:T16)
                  n142 = Bundle By Name(cluster=w315, "alias"=w306, "Config Pane Only"=w311, "Show Term"=w310, "value"=w312) -> (w314:T16)
                  n143 = in-place-array #3(w314, w307) -> (w297:T15)  [unwired: 2 out]
                }
                n144 = in-place-cluster #2("Inputs"=w297) -> (w287:T6)
              }
              n145 = in-place {
                in-place-border: w292 -> [w318]
                n146 = in-place-cluster #4(w294) -> ("Inputs"=w319:T15)
                n147 = in-place {
                  in-place-border: w318 -> [w320]
                  n148 = in-place-array #5(w319, 0) -> (w323:T16)
                  n149 = To Variant(anything=w320) -> (Variant=w321:variant)
                  n150 = Bundle By Name(cluster=w323, "value"=w321) -> (w322:T16)
                  n151 = in-place-array #5(w322) -> (w317:T15)  [unwired: 1 out]
                }
                n152 = in-place-cluster #4("Inputs"=w317) -> (w293:T6)
              }
              n153 = in-place-array #1(w293, w287) -> (w274:T5)  [unwired: 2 out]
            }
            n154 = call <vilib>:"Parse Property Bundle.vi"("Name"="Pin Annotation" ("x"), "Property Bundle"=w227) -> ("Value"=w231:variant)  [unwired: 8 in, 1 out]
            n155 = Variant To Data(type=string[] [], Variant=w231) -> (data=w232:string[])  [unwired: 1 in, 1 out]
            n156 = Index Array(array=w232) -> (element=w225:string)  [unwired: 1 in]
            n157 = Match Pattern(string=w228, regular expression="/") -> (before substring=w236:string, after substring=w239:string)  [unwired: 1 in, 2 out]
            n158 = call <vilib>:"Trim Whitespace.vi"("string"=w239) -> ("trimmed string"=w240:string)  [unwired: 1 in]
            n159 = Match Pattern(string=w225, regular expression="(") -> (after substring=w222:string)  [unwired: 1 in, 3 out]
            n160 = Concatenate Strings("Connector " ("string"), w236) -> (w237:string)
            n161 = Match Pattern(string=w222, regular expression=")") -> (before substring=w221:string)  [unwired: 1 in, 3 out]
            n162 = Bundle By Name(cluster=T14 {"Connector"="", "Alias Name"="", "PIN ID"=""} ("Connection Information"), "Connector"=w237, "Alias Name"=w240, "PIN ID"=w221) -> (w234:T14)
            n163 = Build Array(w234) -> (→"_Connection Informations":T17)
            n164 = Equal?(x="_Default Alias String", y="Name:") -> (x = y?=w266:bool)
            n165 = Select(t="_VI Default Name (Edit and make value default)", s=w266, f="Name:") -> (s? t:f=w265:string)
            n166 = Bundle By Name(cluster=T9 {"Title"="", "Description"="", "icon image path (.bmp)"=path "", "Help Link"="", "WireThrough Terminal Names"={"WireThrough Top In"="", "WireThrough Bottom In"="", "WireThrough Top Out"="", "WireThrough Bottom Out"=""}, "Instrument Driver Method Descriptor Array"=[]} ("Scripter Input"), "Instrument Driver Method Descriptor Array"=w274, "WireThrough Terminal Names"="_WireThrough Info (Edit and make value default)", "Title"=w265, "Description"="" ("Title")) -> (→"_Scripter Input":T9)
          }
          event "Channel:": Value Change {
            n167 = event-data() -> ("NewVal"=w325:u16)  [unwired: 1 in, 3 out]
            n168 = property on="Name:" class="Str"() -> ("Text.Text"=w338:string)  [unwired: 2 in, 2 out]
            n169 = Index Array(array=w326, index=w325) -> (element=w324:string)
            n170 = property on="-Channel Details:" class="Str"("Value"=w324) -> ()  [unwired: 2 in, 2 out]
            n171 = global read "Express VI Framework Strings Global.vi" "Status Message.Invalid Data.Invalid Frequency"() -> (w328:string)
            n172 = local read "_Default Alias String"() -> (w336:string)
            n173 = Search 1D Array(1D array=w335, element=w338) -> (index of element=w341:i32)  [unwired: 1 in]
            n174 = property on="Frequency Unit" class="Enum (strict)"() -> ("Value"=w332:enum16{"Hz", "kHz"})  [unwired: 2 in, 2 out]
            n175 = property on="Frequency:" class="DigNum (strict)"() -> ("Value"=w331:dbl)  [unwired: 2 in, 2 out]
            n176 = Not Equal?(x=w341, y=-1) -> (x != y?=w339:bool)
            n177 = call <vilib>:"PWM Coerce Frequency.vi"("Frequency"=w331, "Frequency Units"=w332) -> ("Coercion needed?"=w330:bool)  [unwired: 8 in, 1 out]
            n178 = Select(t=w336, s=w339, f=w338) -> (s? t:f=w337:string)
            n179 = Not(x=w330) -> (.not. x?=w329:bool)
            n180 = property on="Name:" class="Str"("Text.Text"=w337) -> ()  [unwired: 2 in, 2 out]
            n181 = Bundle By Name(cluster=cluster{"Valid":bool, "Invalid Info":string} {"Valid"=FALSE, "Invalid Info"=""} ("event data"), "Valid"=w329, "Invalid Info"=w328) -> (w333:cluster{"Valid":bool, "Invalid Info":string})
            n182 = Generate User Event(user event=w327, event data cluster=w333) -> ()  [unwired: 2 in, 2 out]
          }
        }
      }
      n183 = Unregister For Events(event registration refnum=w130) -> ()  [unwired: 1 in, 1 out]
    }
  }
